vi "Set State.vi"(8 "error in (no error)":errorcluster, 10 "New State In":refnum<class "State.lvclass">, 11 "Door Controller in":refnum<class "Door Controller.lvclass">) -> (0 "error out":errorcluster, 3 "Door Controller out":refnum<class "Door Controller.lvclass">)   [LabVIEW 2020, in "Door Controller.lvlib" / "Door Controller.lvclass"]
uses:
  Door Controller.lvclass
  State/State.lvclass
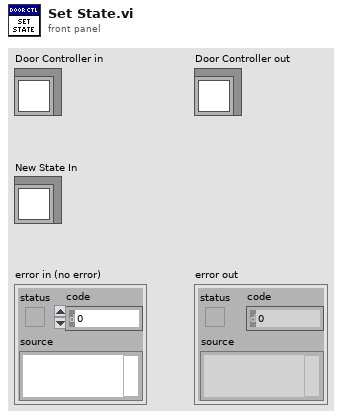
[diagram p1: front panel]
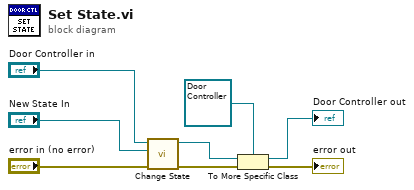
[diagram p0: block diagram]
diagram:
  n1 = call-dynamic "Change State.vi"("error in (no error)"="error in (no error)", "New State In"="New State In", "Door Controller in"="Door Controller in") -> ("error out"=w3:errorcluster, "State Out"=w4:refnum<class "State.lvclass">)  [unwired: 7 in]
  n2 = To More Specific Class(target class=refnum<class "Door Controller.lvclass"> refnum ("Door Controller.lvlib:Door Controller.lvclass"), reference=w4, error in=w3) -> (specific class reference=→"Door Controller out":refnum<class "Door Controller.lvclass">, error out=→"error out":errorcluster)
